vi "Create GCF LUT.vi"(8 "error in (no error)":errorcluster, 11 "FC2901 in":refnum<class "FC2901.lvclass">) -> (0 "error out":errorcluster, 3 "FC2901 out":refnum<class "FC2901.lvclass">)   [LabVIEW 2021, in "FC2901.lvclass"]
uses:
  FC2901.lvclass
  FC2901.lvclass/FC2901.ctl
  <vilib>/Utility/file.llb/Read Delimited Spreadsheet (string).vi
  <vilib>/BenjaminR/LookUp Table API/LUT.lvclass
  GCF Data.ctl
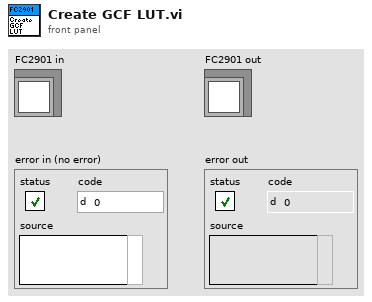
[diagram p1: front panel]
types:
  T1 = typedef "FC2901.lvclass/GCF Data.ctl" = map{string, dbl}
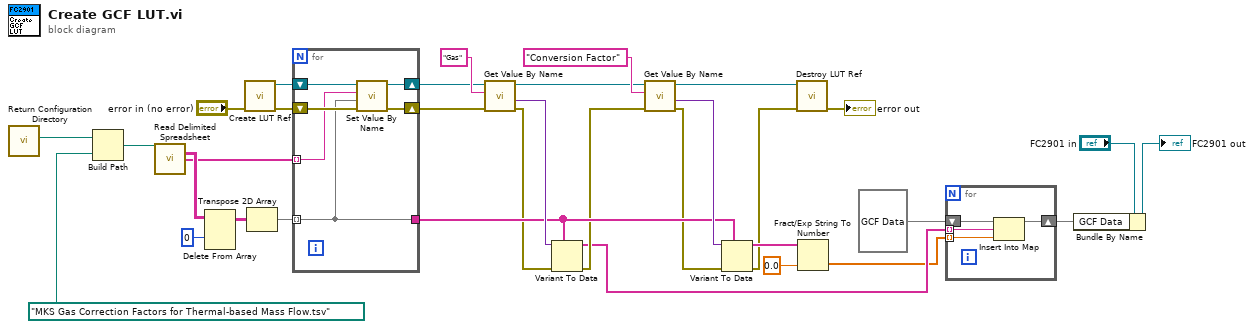
[diagram p0: block diagram]
diagram:
  n1 = call "Return Configuration Directory.vi"() -> ("Configuration Directory"=w1:path)  [unwired: 11 in]
  n2 = Build Path(base path=w1, name or relative path=path "MKS Gas Correction Factors for Thermal-based Mass Flow.tsv" ("file path (dialog if empty)")) -> (appended path=w2:path)
  n3 = call-poly <vilib>:"Read Delimited Spreadsheet.vi"("file path (dialog if empty)"=w2) -> ("all rows"=w33:string[][], "first row"=w30:string[])  [unwired: 9 in, 4 out]
  n4 = Delete From Array(array=w33, index (row)=0) -> (array with subset deleted=w28:string[][])  [unwired: 2 in, 1 out]
  n5 = call <vilib>:"Create LUT Ref.vi"("error in (no error)"="error in (no error)") -> ("error out"=w29:errorcluster, "LUT out"=w31:refnum<class "LUT.lvclass">)  [unwired: 9 in]
  n6 = Transpose 2D Array(2D array=w28) -> (transposed array=w27:string[][])
  n7 = for {
    tunnel: w30 -> [w35] mode=indexing
    tunnel: w27 -> [w34] mode=indexing
    shift-right: [w38] -> w24
    shift-left: w31 -> [w39]
    shift-right: [w37] -> w25
    shift-left: w29 -> [w36]
    tunnel: [w34] -> w19
    n8 = call <vilib>:"Set Value By Name.vi"("error in (no error)"=w36, "Value"=w34, "Name"=w35, "LUT in"=w39) -> ("error out"=w37:errorcluster, "LUT out"=w38:refnum<class "LUT.lvclass">)  [unwired: 5 in, 1 out]
  }
  n9 = call <vilib>:"Get Value By Name.vi"("error in (no error)"=w25, "Name"="Gas", "LUT in"=w24) -> ("error out"=w13:errorcluster, "Value"=w23:variant, "LUT out"=w20:refnum<class "LUT.lvclass">)  [unwired: 5 in, 1 out]
  n10 = Variant To Data(error in=w13, type=w19, Variant=w23) -> (data=w7:string[], error out=w12:errorcluster)
  n11 = call <vilib>:"Get Value By Name.vi"("error in (no error)"=w12, "Name"="Conversion Factor", "LUT in"=w20) -> ("error out"=w11:errorcluster, "Value"=w22:variant, "LUT out"=w16:refnum<class "LUT.lvclass">)  [unwired: 5 in, 1 out]
  n12 = Variant To Data(error in=w11, type=w19, Variant=w22) -> (data=w18:string[], error out=w10:errorcluster)
  n13 = call <vilib>:"Destroy LUT Ref.vi"("error in (no error)"=w10, "LUT in"=w16) -> ("error out"=→"error out":errorcluster)  [unwired: 9 in]
  n14 = Fract/Exp String To Number(string=w18, default (0 dbl)=0.0 ("default (0 DBL)")) -> (number=w6:dbl[])  [unwired: 2 in, 1 out]
  n15 = for {
    tunnel: w7 -> [w43] mode=indexing
    tunnel: w6 -> [w42] mode=indexing
    shift-right: [w40] -> w9
    shift-left: T1 {} ("GCF Data") -> [w41]
    n16 = Insert Into Map(map in=w41, key=w43, value=w42) -> (map out=w40:T1)  [unwired: 2 out]
  }
  n17 = Bundle By Name(cluster="FC2901 in", "GCF Data"=w9) -> (→"FC2901 out":refnum<class "FC2901.lvclass">)
